vi "Load Anything.vi"(0 "Anything":variant, 1 "Path (dialog)":path, 3 "Instance Name":string, 5 "Error In":errorcluster) -> (14 "Data":variant, 19 "error out":errorcluster)   [LabVIEW 2012]
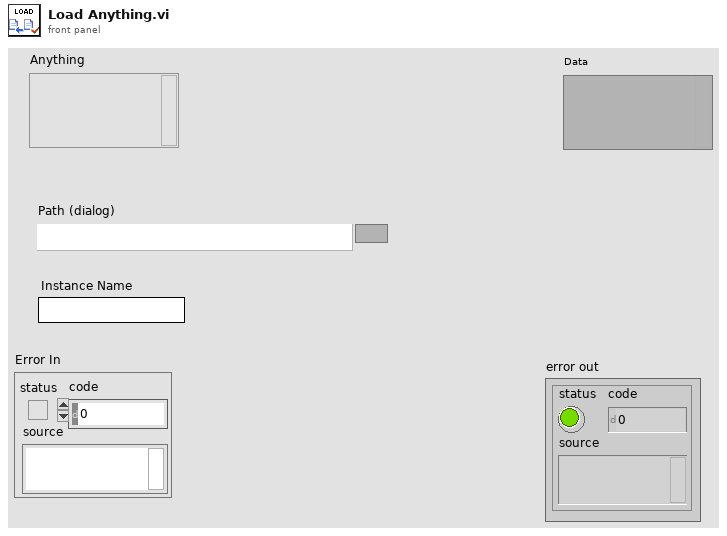
[diagram p1: front panel]
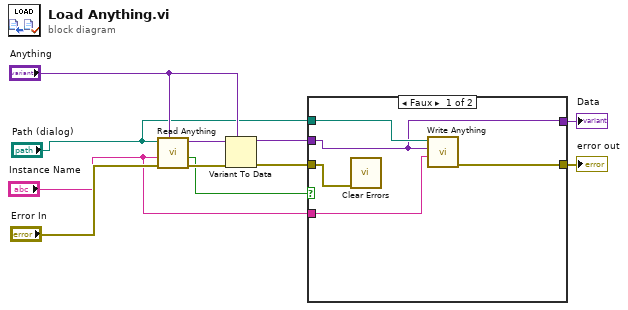
[diagram p0: block diagram]
diagram:
  n1 = call "Read Anything.vi"("Type of Anything"="Anything", "Error In"="Error In", "Section Name (Name of \"Type of Anything\")"="Instance Name", "Path (dialog)"="Path (dialog)") -> ("Error Out"=w9:errorcluster, "Found?"=w7:bool, "Anything"=w8:variant)  [unwired: 5 in]
  n2 = Variant To Data(error in=w9, type="Anything", Variant=w8) -> (data=w5:variant, error out=w6:errorcluster)
  n3 = case shown="Faux" w7 {
    tunnel: w6 -> [w12 w17]
    tunnel: w5 -> [w13 w18]
    tunnel: [w13 w18] -> w4
    tunnel: "Path (dialog)" -> [w16 _]
    tunnel: "Instance Name" -> [w15 _]
    tunnel: [w14 w17] -> w1
    frame False {
      n4 = call <vilib>:"Clear Errors.vi"("error in (no error)"=w12) -> ()  [unwired: 6 in, 1 out]
      n5 = call "Write Anything.vi"("Section Name (Name of \"Anything\")"=w15, "Anything"=w13, "Path (dialog)"=w16) -> ("Error Out"=w14:errorcluster)  [unwired: 8 in]
    }
    frame True {
    }
  }
  "Data" <- w4
  "error out" <- w1
